vi "Get Source Power Span.vi"(8 "error in (no error)":errorcluster {"code" format="%.0x"}, 9 "PortVal":i32 format="%.0g", 10 "Channel":string, 11 "instrument handle":refnum<k15>) -> (0 "error out":errorcluster {"code" format="%.0x"}, 2 "Span":dbl, 3 "instrument handle out":refnum<k15>)   [LabVIEW 2014, in "Agilent NA.lvlib"]
doc: "Sets/Get the power sweep span power"
uses:
  Agilent NA.lvlib
  AgNA.dll
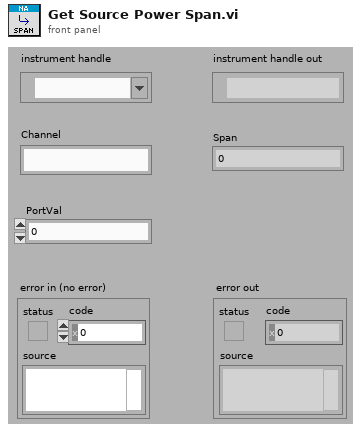
[diagram p1: front panel]
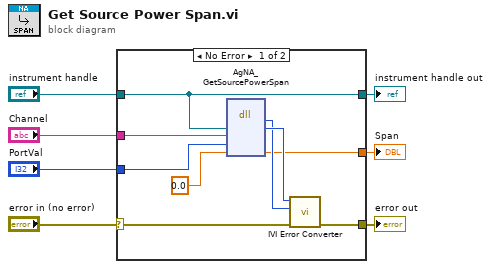
[diagram p0: block diagram]
diagram:
  n1 = case shown="No Error" "error in (no error)" {
    selector: "error in (no error)" -> [w14 w18]
    tunnel: [w13 w18] -> w7
    tunnel: "Channel" -> [w12 _]
    tunnel: "PortVal" -> [w11 _]
    tunnel: [w9 _] -> w3
    tunnel: [w8 w17] -> w2
    tunnel: "instrument handle" -> [w8 w17]
    frame No Error {
      n2 = dll-call lib="AgNA**.dll" fn="AgNA_GetSourcePowerSpan"("Vi"=w8, "Channel"=w12, "PortVal"=w11, "Span"=0.0) -> (w15:i32, "Vi"=w16:u32, "Span"=w9:dbl)  [unwired: 5 in, 2 out]
      n3 = call "IVI Error Converter.vi"("error in (no error)"=w14, "IVI error code (0)"=w15, "instrument handle"=w16) -> ("error out"=w13:errorcluster)  [unwired: 7 in, 1 out]
    }
    frame Error {
    }
  }
  "error out" <- w7
  "instrument handle out" <- w2
  "Span" <- w3
